vi "GenerateWebSocketClientKey.vi"() -> (3 "WebSocket Key":string)   [LabVIEW 2021, in "WebSockets.lvlib" / "WebSocket Client.lvclass"]
doc: "Generates a random string of 16 ASCII characters (from ASCII 37 to 127) for the Sec-WebSocket-Key.\nWebSockets 2.0.1.40\nSam Sharp - MediaMongrels Ltd\nCopyright (c) 2019, MediaMongrels Ltd"
uses:
  WebSocket Client.lvclass
  WebSocket/WebSocket.lvclass
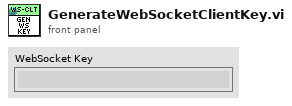
[diagram p1: front panel]
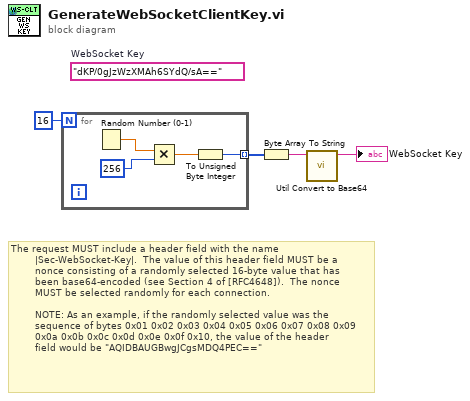
[diagram p0: block diagram]
diagram:
  (unwired) "dKP/0gJzWzXMAh6SYdQ/sA=="  # WebSocket Key
  # "The request MUST include a header field with the name\n        |Sec-WebSocket-Key|.  The value of this header field MUST be a\n        nonce consisting of a randomly selected 16-byte value that has\n        been base64-encoded (see Section 4 of [RFC4648]).  The nonce\n        MUST be selected randomly for each connection.\n\n        NOTE: As an example, if the randomly selected value was the\n        sequence of bytes 0x01 0x02 0x03 0x04 0x05 0x06 0x07 0x08 0x09\n        0x0a 0x0b 0x0c 0x0d 0x0e 0x0f 0x10, the value of the header\n        field would be \"AQIDBAUGBwgJCgsMDQ4PEC==\""
  n1 = for {
    N: 16 -> [_]
    tunnel: [w8] -> w3 mode=indexing
    n2 = Random Number (0-1)() -> (number: 0 to 1=w7:dbl)
    n3 = Multiply(x=w7, y=256) -> (x*y=w5:dbl)
    n4 = To Unsigned Byte Integer(number=w5) -> (unsigned 8bit integer=w8:u8)
  }
  n5 = Byte Array To String(unsigned byte array=w3) -> (string=w2:string)
  n6 = call "Util Convert to Base64.vi"("String"=w2) -> ("Base64 String"=→"WebSocket Key":string)  [unwired: 10 in]
